vi "Errorbar.vi"(4 "Properties":T1={"Color"=2147483647, "Line Width"=nan, "Cap Size"=nan, "Display"={"Alpha"=nan, "Z Order"=nan}} {"Color" items=["Automatic"=2147483647, "Black"=0, "White"=16777215, "Red"=16711680, "Green"=2263842, "Blue"=255, "Cyan"=65535, "Magenta"=16711935, "Yellow"=16776960]}, 5 "Y Errors":dbl[](array[numeric]), 7 "X Errors":dbl[](array[numeric]), 8 "error in (no error)":errorcluster, 9 "Y Data":dbl[](array[numeric]), 10 "X Data":dbl[](array[numeric]), 11 "Plot ID":T4 format="%x") -> (0 "error out":errorcluster, 3 "Plot ID out":T4 format="%x")   [LabVIEW 2013, in "Advanced Plotting Toolkit.lvlib"]
doc: "Overlay error bars on a plot. Note this VI only adds the error bars; use e.g. Line.vi, Scatter.vi or Bar.vi first to plot the actual data."
uses:
  Advanced Plotting Toolkit.lvlib
  typedefs/PlotID.ctl
  ErrorbarProperties.ctl
  typedefs/PlotColor.ctl
  properties/Display.ctl
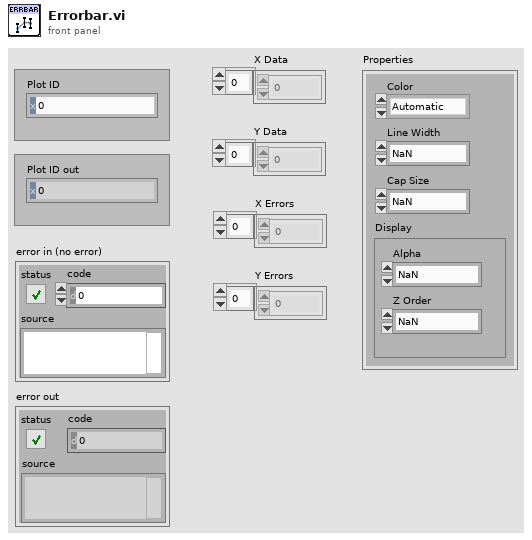
[diagram p1: front panel]
types:
  T1 = typedef "Advanced Plotting Toolkit.lvlib/ErrorbarProperties.ctl" = cluster{"Color":T2, "Line Width":dbl, "Cap Size":dbl, "Display":T3}
  T2 = typedef "Advanced Plotting Toolkit.lvlib/PlotColor.ctl" = u32
  T3 = typedef "Advanced Plotting Toolkit.lvlib/Display.ctl" = cluster{"Alpha":dbl, "Z Order":dbl}
  T4 = typedef "Advanced Plotting Toolkit.lvlib/PlotID.ctl" = i32
  T5 = typedef "Advanced Plotting Toolkit.lvlib/KeyValue.ctl" = cluster{"Key":string, "Value":string}
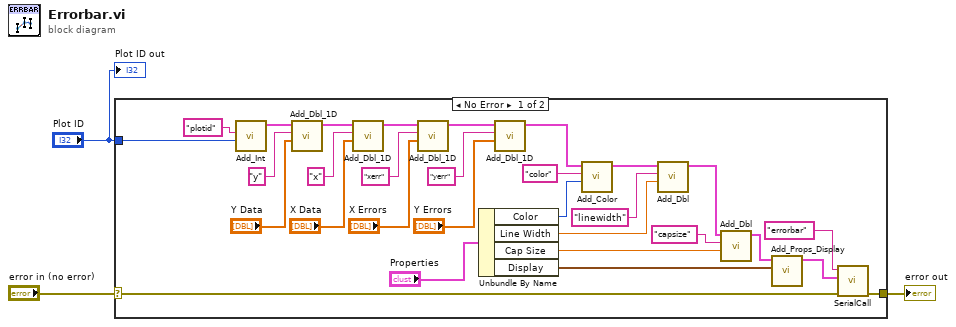
[diagram p0: block diagram]
diagram:
  n1 = case shown="No Error" "error in (no error)" {
    selector: "error in (no error)" -> [w24 w34]
    tunnel: [w31 w34] -> w3
    tunnel: "Plot ID" -> [w21 _]
    frame No Error {
      n2 = call "Add_Int.vi"("Value"=w21, "Key"="plotid" ("Keyword")) -> ("Keyword Array Out"=w30:T5[])  [unwired: 9 in]
      n3 = call "Add_Dbl_1D.vi"("Value"="Y Data", "Key"="y", "Keyword Array"=w30) -> ("Keyword Array Out"=w28:T5[])  [unwired: 8 in]
      n4 = call "Add_Dbl_1D.vi"("Value"="X Data", "Key"="x", "Keyword Array"=w28) -> ("Keyword Array Out"=w20:T5[])  [unwired: 8 in]
      n5 = call "Add_Dbl_1D.vi"("Value"="X Errors", "Key"="xerr", "Keyword Array"=w20) -> ("Keyword Array Out"=w19:T5[])  [unwired: 8 in]
      n6 = Unbundle By Name("Properties") -> ("Color"=w12:T2, "Line Width"=w11:dbl, "Cap Size"=w9:dbl, "Display"=w4:T3)
      n7 = call "Add_Dbl_1D.vi"("Value"="Y Errors", "Key"="yerr", "Keyword Array"=w19) -> ("Keyword Array Out"=w14:T5[])  [unwired: 8 in]
      n8 = call "Add_Color.vi"("Color"=w12, "Key"="color", "Keyword Array"=w14) -> ("Keyword Array Out"=w10:T5[])  [unwired: 8 in]
      n9 = call "Add_Dbl.vi"("Value"=w11, "Key"="linewidth", "Keyword Array"=w10) -> ("Keyword Array Out"=w8:T5[])  [unwired: 8 in]
      n10 = call "Add_Dbl.vi"("Value"=w9, "Key"="capsize", "Keyword Array"=w8) -> ("Keyword Array Out"=w5:T5[])  [unwired: 8 in]
      n11 = call "Add_Props_Display.vi"("Display"=w4, "Keyword Array"=w5) -> ("Keyword Array Out"=w6:T5[])  [unwired: 9 in]
      n12 = call "SerialCall.vi"("error in (no error)"=w24, "data"=w6, "Resource"="errorbar") -> ("error out"=w31:errorcluster)  [unwired: 7 in, 1 out]
    }
    frame Error {
    }
  }
  "error out" <- w3
  "Plot ID out" <- "Plot ID"
